vi "xy振镜移动-v2.1.vi"(0 "AO通道：X前Y后":tag="Dev1/ao0:1", 1 "f_scanlens(mm)":dbl=50.0, 2 "f_tubelens(mm)":dbl=200.0, 3 "f_objecitve(mm)":dbl=1.8, 4 "比例因子(V/°)":dbl=0.5, 5 "x终止位(um)":dbl=10.0, 7 "y终止位(um)":dbl=10.0, 9 "x初始位(um)":dbl, 11 "y初始位(um)":dbl, 12 "速度(um/s)":dbl=10.0) -> (6 "x终止位(um) 2":dbl=10.0, 8 "y终止位(um) 2":dbl=10.0)   [LabVIEW 2015]
doc: "速度为0时执行G0指令，可无需连接XY初始角"
uses:
  <vilib>/Platform/TimedLoop/XDataNode/timing_clust.ctl
  <vilib>/Platform/TimedLoop/XDataNode/nitl_modes.ctl
  <vilib>/Platform/TimedLoop/XDataNode/wakeup.ctl
  <vilib>/DAQmx/write.llb/DAQmx Write (Analog 1D DBL NChan 1Samp).vi
  <vilib>/DAQmx/write.llb/DAQmx Write (Analog DBL 1Chan 1Samp).vi
  <vilib>/DAQmx/create/channels.llb/DAQmx Create Channel (AO-Voltage-Basic).vi
  <vilib>/DAQmx/miscellaneous.llb/DAQmx Fill In Error Info.vi
  <vilib>/Platform/TimedLoop/XDataNode/XDataNode.xnode
  <vilib>/Platform/TimedLoop/XDataNode/XDNodeRunTimeDep.lvlib
panel:
  out "y变压轨迹(°)":dbl[](array[numeric])=[0.0, 0.0, 0.002017457026776073, 0.006052371120349187, 0.012104742510839941, 0.020174571918626052, 0.030261861004579515, 0.042366612970385624, 0.05648883330894886, 0.07262853070489507, 0.09078571808518568, 0.11096041381986907, 0.13315264307300606, 0.15736243930382154, 0.1835898459181542, 0.21183491807029903, 0.24209772461536572, 0.27437835021230905, 0.30867689757782557, 0.3449934898913579, 0.38332827335149355, 0.42368141988411046, 0.46605313000267945, 0.5104436358212108, 0.5568532042204127, 0.6052821401677164, 0.6557307901919239, 0.7081995460133446, 0.7626888483303975, 0.819199190763796, 0.8777311239595615, 0.9382852598522744, 1.0008622760901253, 1.0654629206235144, 1.1320880164591356, 1.2007384665816805, 1.271415259045531, 1.3441194722390282, 1.4188522803241743, 1.495614958854875, 1.5744088905771372, 1.6552355714149243, 1.7380966166457146, 1.8229937672701457, 1.909928896580496, 1.998904016933165, 2.0899212867307106, 2.18298301761946, 2.2780916819091943, 2.375249920221874, 2.4744605493769543, 2.575726570521373, 2.6790511775129087, 2.784437765566249, 2.891889940171799, 3.0014115262979684, 3.1130065778884597, 3.226679387666904, 3.3424344972620594, 3.4602767076677168, 3.5802110900524586, 3.702242996935469, 3.826378073745729, 3.952622270783123, 4.080981855601287, 4.211463425833395, 4.344073922483553, 4.478820643708048, 4.615711259112385, 4.754753824591847, 4.895956797745277, 5.039329053893832, 5.18487990273871, 5.3326191056942776, 5.4825568939355716, 5.6347039872019975, 5.789071613401982, 5.94567152906667, 6.1045160407041665, 6.265618027109712, 6.428990962691198, 6.5946489418739285, 6.762606704653315, 6.932879663369455, 7.105483930783171, 7.2804363495393325, 7.4577545231099505, 7.6374568483168614, 7.819562549541885, 8.004091714740943, 8.19106533338831, 8.380505336487511, 8.572434638796867, 8.766877183430273, 8.963857989007577, 9.163403199544092, 9.365540137285489, 9.570297358712834, 9.777704713962741, 9.987793409930267, 10.200596077346972, 10.416146842154335, 10.634481401523217, 10.855637104904389, 11.079653040532992, 11.306570127852297, 11.536431216369454, 11.769281191509043, 12.00516708808958, 12.244138212115095, 12.486246271648975, 12.731545517622042, 12.980092895522644, 13.231948209024937, 13.487174296734457, 13.745837223369977, 14.008006486859884, 14.27375524301323, 14.543160549633939, 14.816303632185644, 15.09327017338965, 15.374150629455835, 15.659040576013455, 15.948041087234744, 16.241259152139953, 16.53880813265128, 16.84080826864106, 17.14738723601639, 17.45868076482219, 17.774833325457493, 18.095998892422205, 18.42234179659009, 18.754037678895433, 19.09127456059879, 19.434254048052267, 19.783192693234888, 20.13832353542236, 20.499897854386717, 20.868187171740544, 21.24348554477633, 21.62611220683683, 22.01641462046435, 22.4147720250887]
  out "x变压轨迹(°)":dbl[](array[numeric])=[0.0, 0.0, 0.002017457026776073, 0.006052371120349187, 0.012104742510839941, 0.020174571918626052, 0.030261861004579515, 0.042366612970385624, 0.05648883330894886, 0.07262853070489507, 0.09078571808518568, 0.11096041381986907, 0.13315264307300606, 0.15736243930382154, 0.1835898459181542, 0.21183491807029903, 0.24209772461536572, 0.27437835021230905, 0.30867689757782557, 0.3449934898913579, 0.38332827335149355, 0.42368141988411046, 0.46605313000267945, 0.5104436358212108, 0.5568532042204127, 0.6052821401677164, 0.6557307901919239, 0.7081995460133446, 0.7626888483303975, 0.819199190763796, 0.8777311239595615, 0.9382852598522744, 1.0008622760901253, 1.0654629206235144, 1.1320880164591356, 1.2007384665816805, 1.271415259045531, 1.3441194722390282, 1.4188522803241743, 1.495614958854875, 1.5744088905771372, 1.6552355714149243, 1.7380966166457146, 1.8229937672701457, 1.909928896580496, 1.998904016933165, 2.0899212867307106, 2.18298301761946, 2.2780916819091943, 2.375249920221874, 2.4744605493769543, 2.575726570521373, 2.6790511775129087, 2.784437765566249, 2.891889940171799, 3.0014115262979684, 3.1130065778884597, 3.226679387666904, 3.3424344972620594, 3.4602767076677168, 3.5802110900524586, 3.702242996935469, 3.826378073745729, 3.952622270783123, 4.080981855601287, 4.211463425833395, 4.344073922483553, 4.478820643708048, 4.615711259112385, 4.754753824591847, 4.895956797745277, 5.039329053893832, 5.18487990273871, 5.3326191056942776, 5.4825568939355716, 5.6347039872019975, 5.789071613401982, 5.94567152906667, 6.1045160407041665, 6.265618027109712, 6.428990962691198, 6.5946489418739285, 6.762606704653315, 6.932879663369455, 7.105483930783171, 7.2804363495393325, 7.4577545231099505, 7.6374568483168614, 7.819562549541885, 8.004091714740943, 8.19106533338831, 8.380505336487511, 8.572434638796867, 8.766877183430273, 8.963857989007577, 9.163403199544092, 9.365540137285489, 9.570297358712834, 9.777704713962741, 9.987793409930267, 10.200596077346972, 10.416146842154335, 10.634481401523217, 10.855637104904389, 11.079653040532992, 11.306570127852297, 11.536431216369454, 11.769281191509043, 12.00516708808958, 12.244138212115095, 12.486246271648975, 12.731545517622042, 12.980092895522644, 13.231948209024937, 13.487174296734457, 13.745837223369977, 14.008006486859884, 14.27375524301323, 14.543160549633939, 14.816303632185644, 15.09327017338965, 15.374150629455835, 15.659040576013455, 15.948041087234744, 16.241259152139953, 16.53880813265128, 16.84080826864106, 17.14738723601639, 17.45868076482219, 17.774833325457493, 18.095998892422205, 18.42234179659009, 18.754037678895433, 19.09127456059879, 19.434254048052267, 19.783192693234888, 20.13832353542236, 20.499897854386717, 20.868187171740544, 21.24348554477633, 21.62611220683683, 22.01641462046435, 22.4147720250887]
  out "移动次数":i32=142
  in  "AO通道：单通道":tag="Dev1/ao0:1"
  in  "dt(ms)":i32=10
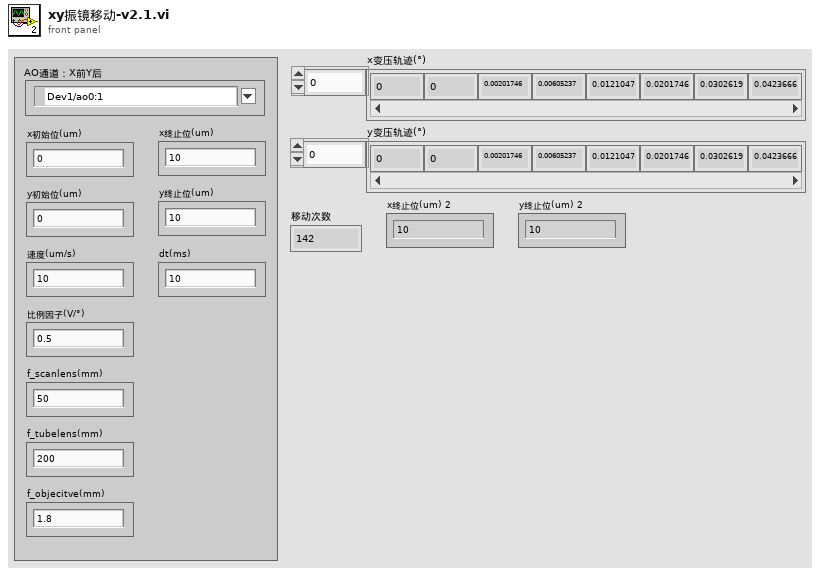
[diagram p1: front panel]
types:
  T1 = typedef "XDNodeRunTimeDep.lvlib/timing_clust.ctl" = cluster{"Expected End [f-1]":u64, "Actual End [f-1]":u64, "Finished Late? [f-1]":bool, "Expected End [i-1]":u64, "Actual End [i-1]":u64, "Finished Late? [i-1]":bool, "Expected Start [i]":u64, "Actual Start [i]":u64, "Expected Start [f]":u64, "Actual Start [f]":u64, "Source Name":string, "Structure Name":string, "Period":i64, "Deadline":i64, "Offset":i64, "Start":i64, "Priority":i32, "Timeout":i32, "Mode":T2, "Wakeup Reason":T3, "Error":errorcluster, "Source Type":string, "Secondary Source Type":string, "Global End Time":u64, "Global Start Time":u64, "Frame Duration":u64, "Iteration Duration":u64, "Assigned CPU":i32, "I/O Scan Engine Mode":u32}
  T2 = typedef "XDNodeRunTimeDep.lvlib/nitl_modes.ctl" = enum32{"No Change", "Process missed periods, maintain original phase", "Discard missed periods, maintain original phase", "Process missed periods, ignore original phase", "Discard missed periods, ignore original phase"}
  T3 = typedef "XDNodeRunTimeDep.lvlib/wakeup.ctl" = enum32{"Normal", "Aborted", "Asynchronous wakeup", "Timing source error", "Timed loop error", "Timeout"}
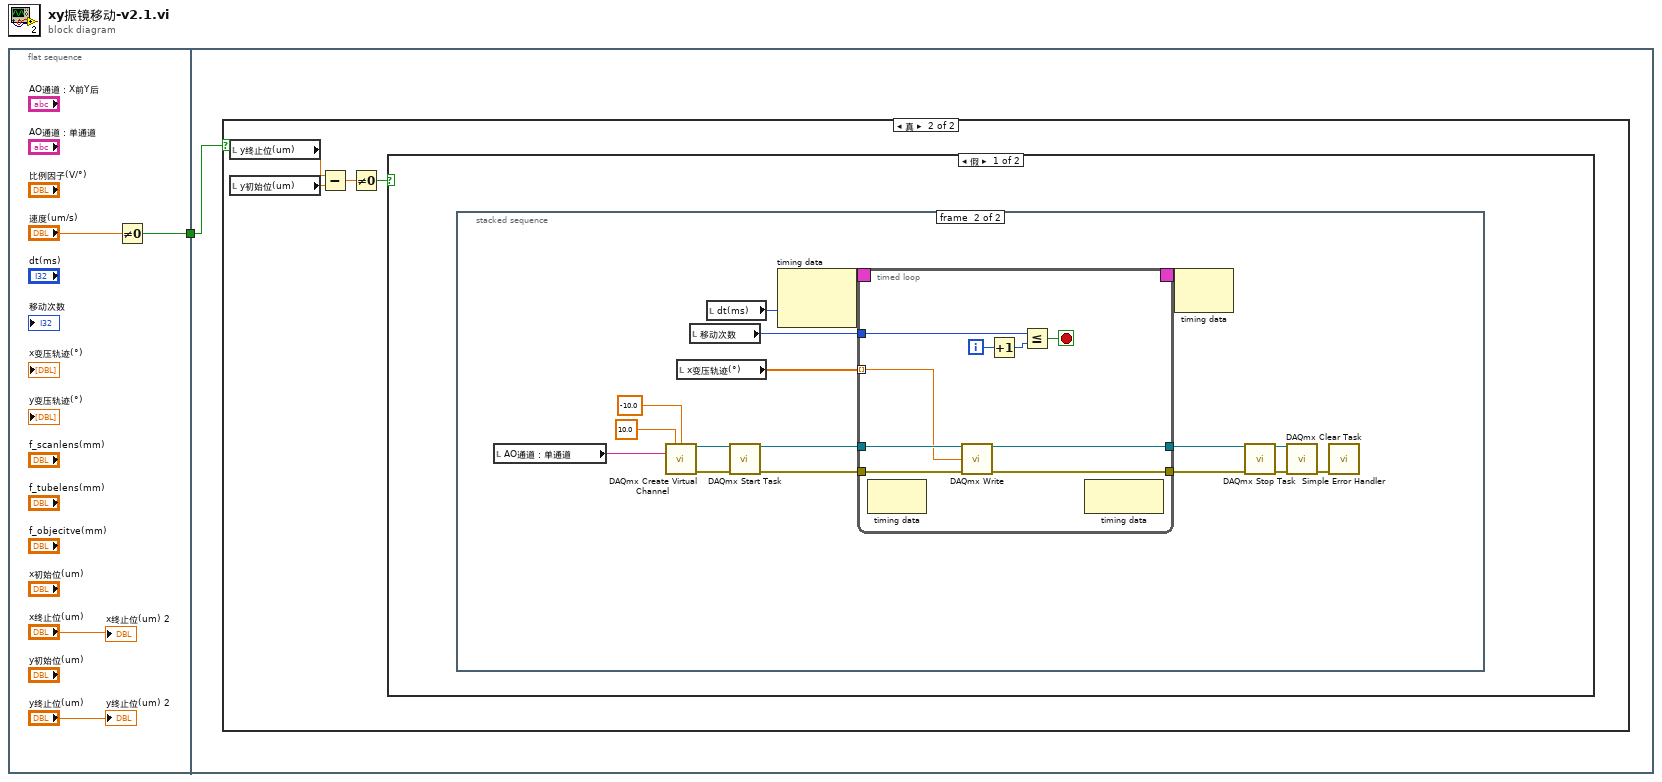
[diagram p0: block diagram]
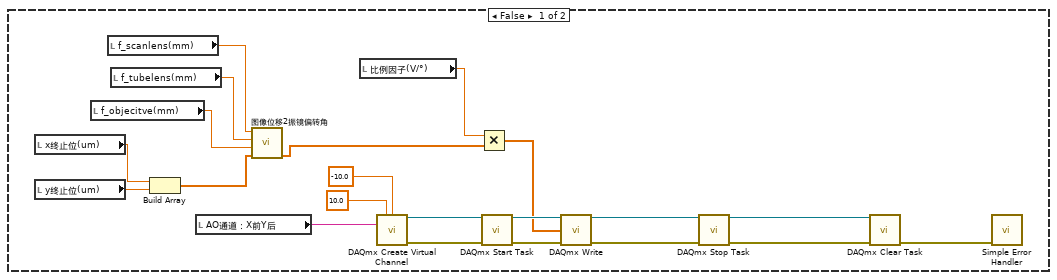
[diagram p2: hidden frame]
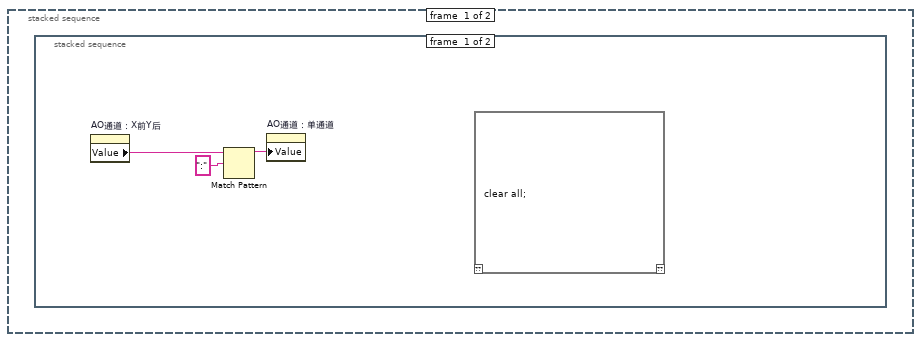
[diagram p3: hidden frame]
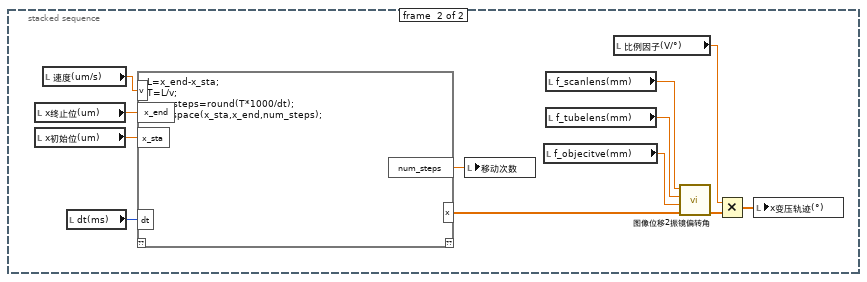
[diagram p4: hidden frame]
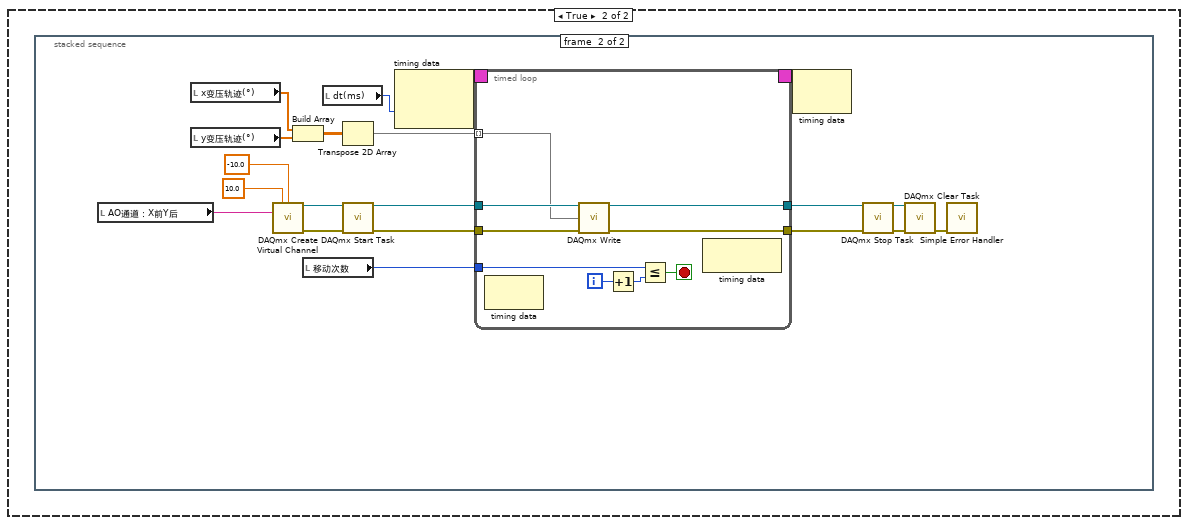
[diagram p5: hidden frame]
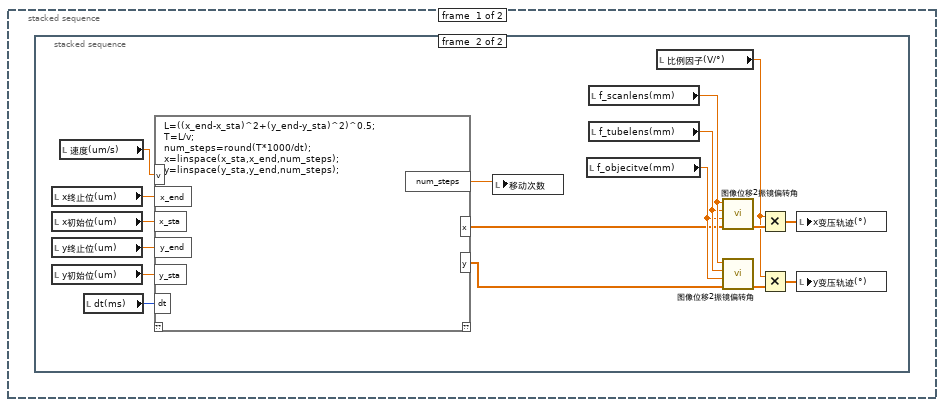
[diagram p6: hidden frame]
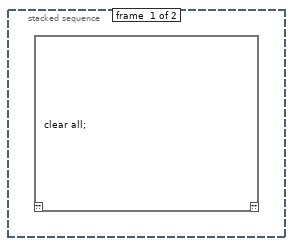
[diagram p7: hidden frame]
diagram:
  n1 = flat-sequence {
    tunnel: [w5] -> w1
    tunnel: w1 -> [w6]
    frame #0 {
      n2 = Not Equal To 0?(x="速度(um/s)") -> (x != 0?=w5:bool)
      "x终止位(um) 2" <- "x终止位(um)"
      "y终止位(um) 2" <- "y终止位(um)"
    }
    frame #1 {
      n3 = case shown="真" w6 {
        frame False {
          n4 = local read "x终止位(um)"() -> (w14:dbl)
          n5 = local read "y终止位(um)"() -> (w15:dbl)
          n6 = local read "f_objecitve(mm)"() -> (w9:dbl)
          n7 = local read "f_scanlens(mm)"() -> (w11:dbl)
          n8 = local read "f_tubelens(mm)"() -> (w10:dbl)
          n9 = Build Array(w14, w15) -> (w8:dbl[])
          n10 = local read "AO通道：X前Y后"() -> (w12:tag)
          n11 = call "图像位移2振镜偏转角.vi"("图像位移(um)"=w8, "f_objecitve(mm)"=w9, "f_tubelens(mm)"=w10, "f_scanlens(mm)"=w11) -> ("振镜偏转角(°)"=w7:dbl[])  [unwired: 7 in]
          n12 = local read "比例因子(V/°)"() -> (w13:dbl)
          n13 = call-poly <vilib>:"DAQmx Create Virtual Channel.vi"("maximum value"=10.0, "minimum value"=-10.0, "physical channels"=w12) -> ("task out"=w26:refnum<k21>, "error out"=w25:errorcluster)  [unwired: 11 in]
          n14 = Multiply(x=w13, y=w7) -> (x*y=w19:dbl[])
          n15 = call <vilib>:"DAQmx Start Task.vi"("task/channels in"=w26, "error in"=w25) -> ("task out"=w20:refnum<k21>, "error out"=w16:errorcluster)  [unwired: 12 in]
          n16 = call-poly <vilib>:"DAQmx Write.vi"("task/channels in"=w20, "data"=w19, "error in"=w16) -> ("task out"=w18:refnum<k21>, "error out"=w17:errorcluster)  [unwired: 10 in, 1 out]
          n17 = call <vilib>:"DAQmx Stop Task.vi"("task/channels in"=w18, "error in"=w17) -> ("task out"=w24:refnum<k21>, "error out"=w23:errorcluster)  [unwired: 12 in]
          n18 = call <vilib>:"DAQmx Clear Task.vi"("task in"=w24, "error in"=w23) -> ("error out"=w27:errorcluster)  [unwired: 13 in]
          n19 = call <vilib>:"Simple Error Handler.vi"("error in (no error)"=w27) -> ()  [unwired: 4 in, 5 out]
        }
        frame True {
          n20 = local read "y终止位(um)"() -> (w29:dbl)
          n21 = local read "y初始位(um)"() -> (w28:dbl)
          n22 = Subtract(x=w29, y=w28) -> (x-y=w31:dbl)
          n23 = Not Equal To 0?(x=w31) -> (x != 0?=w30:bool)
          n24 = case shown="假" w30 {
            frame False {
              n25 = stacked-sequence {
                frame #0 {
                  n26 = stacked-sequence {
                    frame #0 {
                      n27 = property on="AO通道：X前Y后" class="DAQmxName"() -> ("Value"=w34:string)  [unwired: 2 in, 2 out]
                      n28 = Match Pattern(string=w34, regular expression=":" ("正则表达式")) -> (before substring=w32:string)  [unwired: 1 in, 3 out]
                      n29 = property on="AO通道：单通道" class="DAQmxName"("Value"=w32) -> ()  [unwired: 2 in, 2 out]
                      n30 = script code="clear all;"() -> ()  [unwired: 1 in, 1 out]
                    }
                    frame #1 {
                      n31 = local read "x终止位(um)"() -> (w40:dbl)
                      n32 = local read "x初始位(um)"() -> (w39:dbl)
                      n33 = local read "速度(um/s)"() -> (w38:dbl)
                      n34 = local read "dt(ms)"() -> (w37:i32)
                      n35 = script code="L=x_end-x_sta;\nT=L/v;\nnum_steps=round(T*1000/dt);\nx=linspace(x_sta,x_end,num_steps);"("x_sta"=w39, "x_end"=w40, "v"=w38, "dt"=w37) -> ("x"=w35:dbl[], "num_steps"=w36:dbl)  [unwired: 1 in, 1 out]
                      n36 = local write "移动次数"(w36) -> ()
                      n37 = local read "f_objecitve(mm)"() -> (w43:dbl)
                      n38 = local read "f_scanlens(mm)"() -> (w41:dbl)
                      n39 = local read "f_tubelens(mm)"() -> (w42:dbl)
                      n40 = local read "比例因子(V/°)"() -> (w46:dbl)
                      n41 = call "图像位移2振镜偏转角.vi"("图像位移(um)"=w35, "f_objecitve(mm)"=w43, "f_tubelens(mm)"=w42, "f_scanlens(mm)"=w41) -> ("振镜偏转角(°)"=w44:dbl[])  [unwired: 7 in]
                      n42 = Multiply(x=w46, y=w44) -> (x*y=w45:dbl[])
                      n43 = local write "x变压轨迹(°)"(w45) -> ()
                    }
                  }
                }
                frame #1 {
                  n44 = local read "AO通道：单通道"() -> (w49:tag)
                  n45 = call-poly <vilib>:"DAQmx Create Virtual Channel.vi"("maximum value"=10.0, "minimum value"=-10.0, "physical channels"=w49) -> ("task out"=w60:refnum<k21>, "error out"=w59:errorcluster)  [unwired: 11 in]
                  n46 = local read "x变压轨迹(°)"() -> (w47:dbl[])
                  n47 = local read "移动次数"() -> (w48:i32)
                  n48 = local read "dt(ms)"() -> (w52:i32)
                  n49 = call <vilib>:"DAQmx Start Task.vi"("task/channels in"=w60, "error in"=w59) -> ("task out"=w58:refnum<k21>, "error out"=w57:errorcluster)  [unwired: 12 in]
                  n50 = node-c288(w52) -> (w63:T1)  [unwired: 1 in]
                  n51 = timed-loop {
                    tunnel: w58 -> [w72]
                    tunnel: w57 -> [w70]
                    tunnel: [w69] -> w55
                    tunnel: [w71] -> w56
                    timing: w63 -> [_]
                    timing-out: [_] -> w62
                    tunnel: w48 -> [w66]
                    tunnel: w47 -> [w64] mode=indexing
                    i -> [w68]
                    stop <- w65 stop-if-true
                    n52 = node-c288() -> ()  [unwired: 1 in, 1 out]
                    n53 = call-poly <vilib>:"DAQmx Write.vi"("task/channels in"=w72, "data"=w64, "error in"=w70) -> ("task out"=w71:refnum<k21>, "error out"=w69:errorcluster)  [unwired: 10 in, 1 out]
                    n54 = Increment(x=w68) -> (x+1=w67:i32)
                    n55 = Less Or Equal?(x=w66, y=w67) -> (x <= y?=w65:bool)
                    n56 = node-c288() -> ()  [unwired: 1 in, 1 out]
                  }
                  n57 = node-c288(w62) -> ()  [unwired: 1 out]
                  n58 = call <vilib>:"DAQmx Stop Task.vi"("task/channels in"=w56, "error in"=w55) -> ("task out"=w54:refnum<k21>, "error out"=w53:errorcluster)  [unwired: 12 in]
                  n59 = call <vilib>:"DAQmx Clear Task.vi"("task in"=w54, "error in"=w53) -> ("error out"=w61:errorcluster)  [unwired: 13 in]
                  n60 = call <vilib>:"Simple Error Handler.vi"("error in (no error)"=w61) -> ()  [unwired: 4 in, 5 out]
                }
              }
            }
            frame True {
              n61 = stacked-sequence {
                frame #0 {
                  n62 = stacked-sequence {
                    frame #0 {
                      n63 = script code="clear all;"() -> ()  [unwired: 1 in, 1 out]
                    }
                    frame #1 {
                      n64 = local read "x终止位(um)"() -> (w87:dbl)
                      n65 = local read "x初始位(um)"() -> (w86:dbl)
                      n66 = local read "y终止位(um)"() -> (w85:dbl)
                      n67 = local read "y初始位(um)"() -> (w84:dbl)
                      n68 = local read "速度(um/s)"() -> (w83:dbl)
                      n69 = local read "dt(ms)"() -> (w82:i32)
                      n70 = script code="L=((x_end-x_sta)^2+(y_end-y_sta)^2)^0.5;\nT=L/v;\nnum_steps=round(T*1000/dt);\nx=linspace(x_sta,x_end,num_steps);\ny=linspace(y_sta,y_end,num_steps);"("x_sta"=w86, "x_end"=w87, "y_sta"=w84, "y_end"=w85, "v"=w83, "dt"=w82) -> ("x"=w81:dbl[], "y"=w80:dbl[], "num_steps"=w79:dbl)  [unwired: 1 in, 1 out]
                      n71 = local write "移动次数"(w79) -> ()
                      n72 = local read "f_objecitve(mm)"() -> (w93:dbl)
                      n73 = local read "f_scanlens(mm)"() -> (w95:dbl)
                      n74 = local read "f_tubelens(mm)"() -> (w94:dbl)
                      n75 = local read "比例因子(V/°)"() -> (w89:dbl)
                      n76 = call "图像位移2振镜偏转角.vi"("图像位移(um)"=w81, "f_objecitve(mm)"=w93, "f_tubelens(mm)"=w94, "f_scanlens(mm)"=w95) -> ("振镜偏转角(°)"=w92:dbl[])  [unwired: 7 in]
                      n77 = call "图像位移2振镜偏转角.vi"("图像位移(um)"=w80, "f_objecitve(mm)"=w93, "f_tubelens(mm)"=w94, "f_scanlens(mm)"=w95) -> ("振镜偏转角(°)"=w90:dbl[])  [unwired: 7 in]
                      n78 = Multiply(x=w89, y=w92) -> (x*y=w91:dbl[])
                      n79 = Multiply(x=w89, y=w90) -> (x*y=w88:dbl[])
                      n80 = local write "x变压轨迹(°)"(w91) -> ()
                      n81 = local write "y变压轨迹(°)"(w88) -> ()
                    }
                  }
                }
                frame #1 {
                  n82 = local read "AO通道：X前Y后"() -> (w101:tag)
                  n83 = local read "x变压轨迹(°)"() -> (w99:dbl[])
                  n84 = local read "y变压轨迹(°)"() -> (w98:dbl[])
                  n85 = call-poly <vilib>:"DAQmx Create Virtual Channel.vi"("maximum value"=10.0, "minimum value"=-10.0, "physical channels"=w101) -> ("task out"=w112:refnum<k21>, "error out"=w111:errorcluster)  [unwired: 11 in]
                  n86 = Build Array(w99, w98) -> (w97:dbl[][])
                  n87 = local read "移动次数"() -> (w100:i32)
                  n88 = local read "dt(ms)"() -> (w104:i32)
                  n89 = Transpose 2D Array(2D array=w97) -> (transposed array=w96:dbl[][])
                  n90 = call <vilib>:"DAQmx Start Task.vi"("task/channels in"=w112, "error in"=w111) -> ("task out"=w110:refnum<k21>, "error out"=w109:errorcluster)  [unwired: 12 in]
                  n91 = node-c288(w104) -> (w115:T1)  [unwired: 1 in]
                  n92 = timed-loop {
                    tunnel: w110 -> [w124]
                    tunnel: w109 -> [w122]
                    tunnel: [w121] -> w107
                    tunnel: [w123] -> w108
                    timing: w115 -> [_]
                    timing-out: [_] -> w114
                    tunnel: w100 -> [w117]
                    tunnel: w96 -> [w116] mode=indexing
                    i -> [w120]
                    stop <- w118 stop-if-true
                    n93 = node-c288() -> ()  [unwired: 1 in, 1 out]
                    n94 = call-poly <vilib>:"DAQmx Write.vi"("task/channels in"=w124, "data"=w116, "error in"=w122) -> ("task out"=w123:refnum<k21>, "error out"=w121:errorcluster)  [unwired: 10 in, 1 out]
                    n95 = Increment(x=w120) -> (x+1=w119:i32)
                    n96 = Less Or Equal?(x=w117, y=w119) -> (x <= y?=w118:bool)
                    n97 = node-c288() -> ()  [unwired: 1 in, 1 out]
                  }
                  n98 = node-c288(w114) -> ()  [unwired: 1 out]
                  n99 = call <vilib>:"DAQmx Stop Task.vi"("task/channels in"=w108, "error in"=w107) -> ("task out"=w106:refnum<k21>, "error out"=w105:errorcluster)  [unwired: 12 in]
                  n100 = call <vilib>:"DAQmx Clear Task.vi"("task in"=w106, "error in"=w105) -> ("error out"=w113:errorcluster)  [unwired: 13 in]
                  n101 = call <vilib>:"Simple Error Handler.vi"("error in (no error)"=w113) -> ()  [unwired: 4 in, 5 out]
                }
              }
            }
          }
        }
      }
    }
  }
